vi "getShootingParameters.vi"(0 "shotTime":dbl, 1 "Turret_Angle_Deg":dbl, 2 "RobotPose":T3={"TRANSLATION"={"X"=0.0, "Y"=0.0}, "ROTATION"={"VALUE"=0.0, "COS"=1.0, "SIN"=0.0}} {"ROTATION"."SIN" format="%13.4f"; "ROTATION"."COS" format="%13.4f"; "ROTATION"."VALUE" format="%13.4f"; "TRANSLATION"."Y" format="%14.3f"; "TRANSLATION"."X" format="%14.3f"}, 3 "TurretToField":T3={"TRANSLATION"={"X"=0.0, "Y"=0.0}, "ROTATION"={"VALUE"=0.0, "COS"=1.0, "SIN"=0.0}} {"ROTATION"."SIN" format="%13.4f"; "ROTATION"."COS" format="%13.4f"; "ROTATION"."VALUE" format="%13.4f"; "TRANSLATION"."Y" format="%14.3f"; "TRANSLATION"."X" format="%14.3f"}, 5 "ShootingGoalPose":T3={"TRANSLATION"={"X"=0.0, "Y"=0.0}, "ROTATION"={"VALUE"=0.0, "COS"=1.0, "SIN"=0.0}} {"ROTATION"."SIN" format="%13.4f"; "ROTATION"."COS" format="%13.4f"; "ROTATION"."VALUE" format="%13.4f"; "TRANSLATION"."Y" format="%14.3f"; "TRANSLATION"."X" format="%14.3f"}, 6 "RobotVelocity":T1, 10 "AllowShootOnMove":bool) -> (9 "shot_speed":dbl, 11 "turret_adjustment":dbl, 13 "turret_error":T2 {"SIN" format="%13.4f"; "COS" format="%13.4f"; "VALUE" format="%13.4f"}, 14 "uncompensated_yaw_angle_deg":dbl, 15 "uncompensated_range_m":dbl, 16 "effective_yaw_angle_deg":dbl, 17 "effective_range_m":dbl, 18 "effective_yaw_feedforward_velocity_deg_s":dbl, 19 "effective_range_feedforward_m_s":dbl)   [LabVIEW 2023]
doc: "getShootingParameters is a stripped code from Team 254 - FRC_2022 repo, and re-implemented in LabVIEW.\n\nReturns the Transform2d that maps the one pose to another.\n\nParameter:\n - shotTime - Average shot time in seconds for a Game Piece traveling from robot to goal.\n - RobotPose - Current Field-To-Robot Pose.\n - Turret_Angle_Deg - Current Turret's absolute angle in degrees.\n - TurretToField - Current Turret-To-Field Pose ( from ([Robot-To-Turret] + [Field-To-Robot]).inverse )\n - ShootingGoalPose - Your Shooting Target Pose (Field-To-Goal)\n - RobotVelocity - Current ChassisSpeeds (vX, vY, vAng) but in Twist2d\n - AllowShootOnMove - Enable ShootOnMove correction\n\nReturns:\n - uncompensated_yaw_angle_deg - Yaw angle setpoint for Turret\n - uncompensated_range_m - Distance between turret and Goal\n - effective_yaw_angle_deg - (ShootOnMove) Yaw angle setpoint for Turret\n - effective_range_m - (ShootOnMove) Distance between turret and Goal\n - effective_yaw_feedforward_velocity_deg_s - FF value for velocity correction (only correction for uncompensated_yaw_angle)\n - effective_range_feedforward_m_s - FF value (TBD)"
uses:
  <vilib>/Rock Robotics/WPI/ThirdParty/JAS_Junk/TrajLib/TypeDef/POSE2D.ctl
  <vilib>/Rock Robotics/WPI/ThirdParty/JAS_Junk/TrajLib/TypeDef/TRANSLATION2D.ctl
  <vilib>/Rock Robotics/WPI/ThirdParty/JAS_Junk/TrajLib/TypeDef/ROTATION2D.ctl
  <vilib>/Rock Robotics/WPI/ThirdParty/JAS_Junk/TrajLib/TypeDef/TRANSFORM2D.ctl
  <vilib>/Rock Robotics/WPI/ThirdParty/JAS_Junk/TrajLib/TypeDef/TWIST2D.ctl
  <vilib>/Rock Robotics/WPI/ThirdParty/JAS_Junk/TrajLib/Conv_Deg_Radians.vi
  <vilib>/Rock Robotics/WPI/ThirdParty/JAS_Junk/TrajLib/Rotation2d_CreateAngle.vi
  <vilib>/Rock Robotics/WPI/ThirdParty/JAS_Junk/TrajLib/Pose2d_RelativeTo.vi
  <vilib>/Rock Robotics/WPI/ThirdParty/JAS_Junk/TrajLib/Pose2d_TransformBy.vi
  <vilib>/Rock Robotics/WPI/ThirdParty/JAS_Junk/TrajLib/Rotation2d_RotateBy.vi
  <vilib>/Rock Robotics/WPI/ThirdParty/JAS_Junk/TrajLib/Rotation2d_GetRadians.vi
  <vilib>/Rock Robotics/WPI/ThirdParty/JAS_Junk/TrajLib/Transform2d_Create_PosePose.vi
  <vilib>/Rock Robotics/WPI/ThirdParty/JAS_Junk/TrajLib/Pose2d_New_TRRO.vi
  <vilib>/Rock Robotics/WPI/ThirdParty/JAS_Junk/TrajLib/Translation2d_Plus.vi
  <vilib>/Rock Robotics/WPI/ThirdParty/JAS_Junk/TrajLib/Translation2d_Minus.vi
  <vilib>/Rock Robotics/WPI/ThirdParty/JAS_Junk/TrajLib/Rotation2d_Minus.vi
  <vilib>/Rock Robotics/WPI/ThirdParty/JAS_Junk/TrajLib/Trajectory_Library.lvlib
panel:
  out "aimingParams.robot_to_goal_rotation":T2 {"SIN" format="%13.4f"; "COS" format="%13.4f"; "VALUE" format="%13.4f"}
  out "aimingParams.range":dbl
  out "RobotToGoal_tf":T5={"TRANSLATION"={"X"=0.0, "Y"=0.0}, "ROTATION"={"VALUE"=0.0, "COS"=1.0, "SIN"=0.0}, "xF"=FALSE} {"ROTATION"."SIN" format="%13.4f"; "ROTATION"."COS" format="%13.4f"; "ROTATION"."VALUE" format="%13.4f"; "TRANSLATION"."Y" format="%14.3f"; "TRANSLATION"."X" format="%14.3f"}
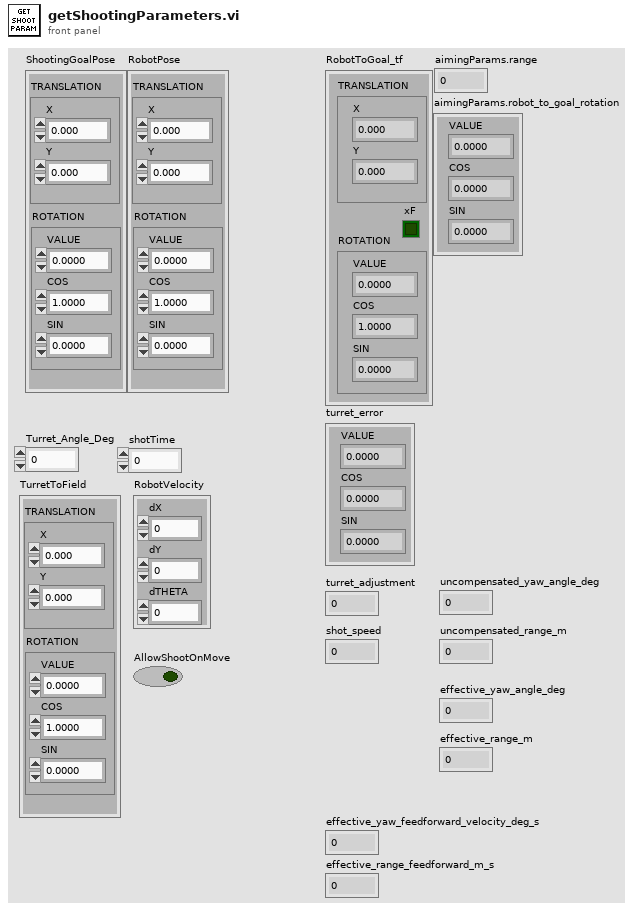
[diagram p1: front panel]
types:
  T1 = typedef "Trajectory_Library.lvlib/TWIST2D.ctl" = cluster{"dX":dbl, "dY":dbl, "dTHETA":dbl}
  T2 = typedef "Trajectory_Library.lvlib/ROTATION2D.ctl" = cluster{"VALUE":dbl, "COS":dbl, "SIN":dbl}
  T3 = typedef "Trajectory_Library.lvlib/POSE2D.ctl" = cluster{"TRANSLATION":T4, "ROTATION":T2}
  T4 = typedef "Trajectory_Library.lvlib/TRANSLATION2D.ctl" = cluster{"X":dbl, "Y":dbl}
  T5 = typedef "Trajectory_Library.lvlib/TRANSFORM2D.ctl" = cluster{"TRANSLATION":T4, "ROTATION":T2, "xF":bool}
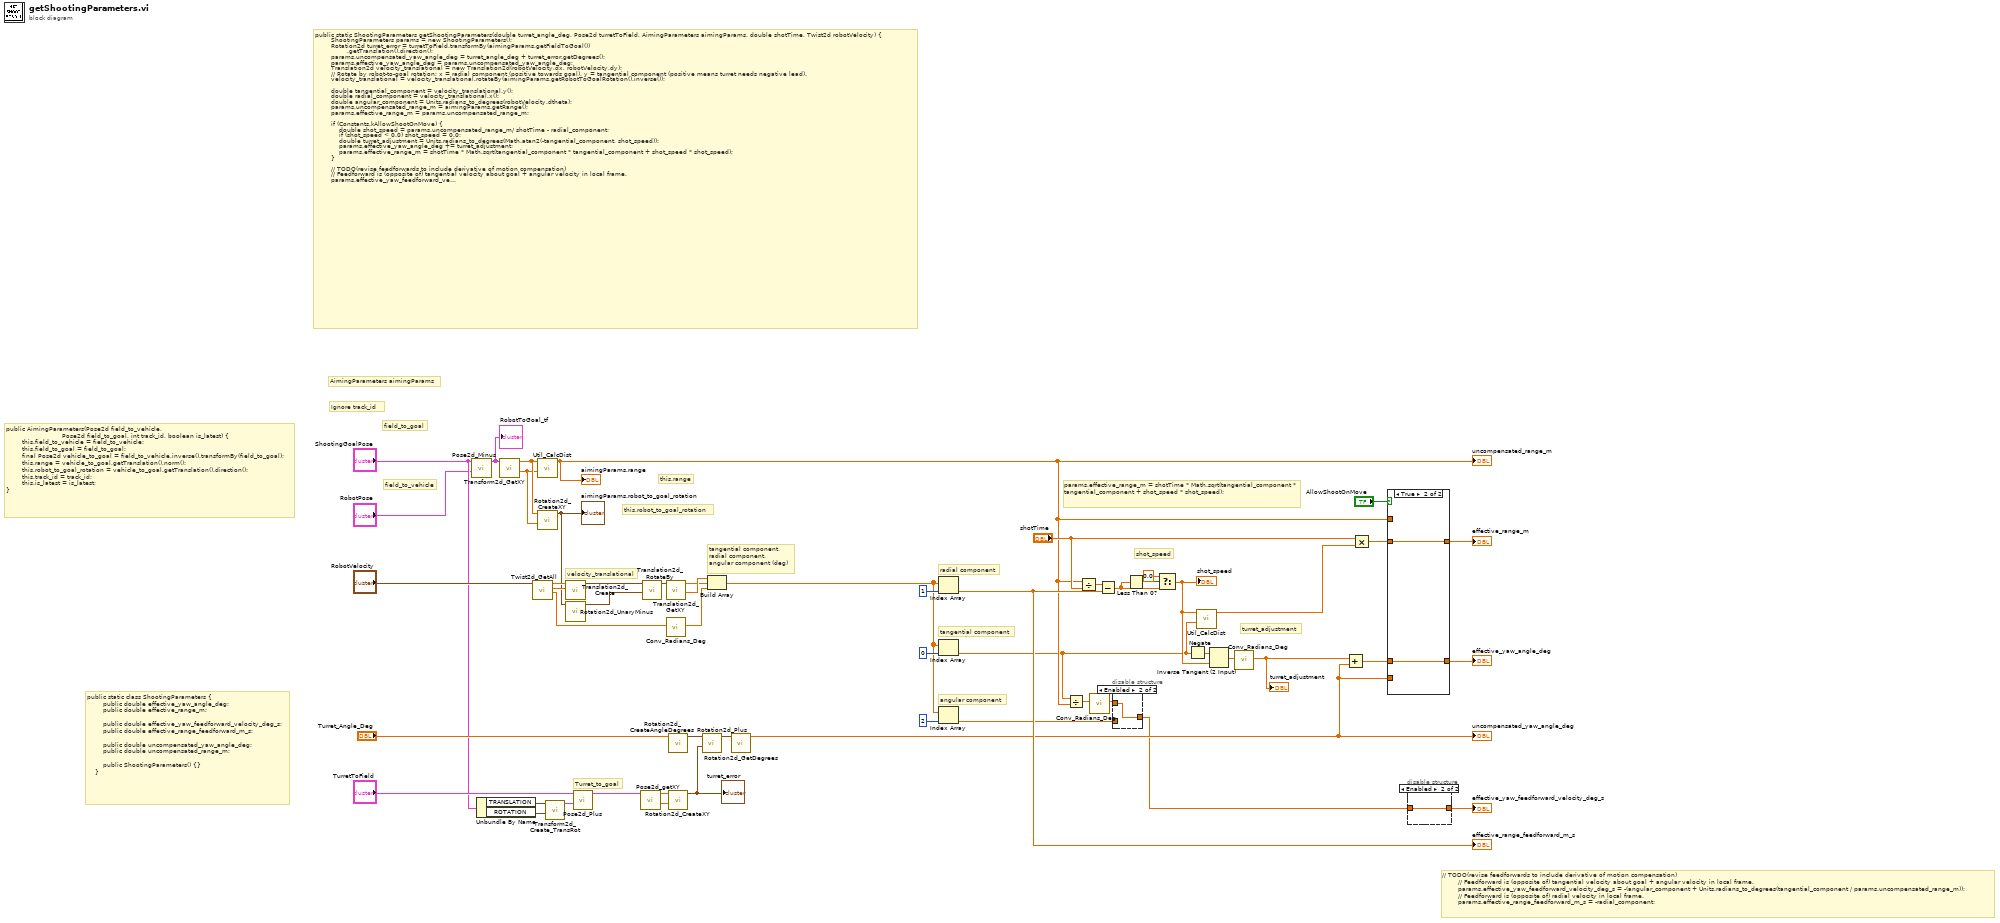
[diagram p0: block diagram]
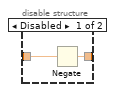
[diagram p2: hidden frame]
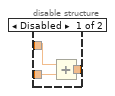
[diagram p3: hidden frame]
diagram:
  # "// TODO(revise feedforwards to include derivative of motion compensation)\n        // Feedforward is (opposite of) tangential velocity about goal + angular velocity in local frame.\n        params.effective_yaw_feedforward_velocity_deg_s = -(angular_component + Units.radians_to_degrees(tangential_component / params.uncompensated_range_m));\n        // Feedforward is (opposite of) radial velocity in local frame.\n        params.effective_range_feedforward_m_s = -radial_component;"
  # "angular component"
  # "radial component"
  # "tangential component"
  # "params.effective_range_m = shotTime * Math.sqrt(tangential_component * tangential_component + shot_speed * shot_speed);"
  # "turret_adjustment"
  # "shot_speed"
  # "tangential component,\nradial component,\nangular component (deg)"
  # "velocity_translational"
  # "Turret_to_goal"
  # "public static class ShootingParameters {\n        public double effective_yaw_angle_deg;\n        public double effective_range_m;\n\n        public double effective_yaw_feedforward_velocity_deg_s;\n        public double effective_range_feedforward_m_s;\n\n        public double uncompensated_yaw_angle_deg;\n        public double uncompensated_range_m;\n\n        public ShootingParameters() {}\n    }"
  # "public static ShootingParameters getShootingParameters(double turret_angle_deg, Pose2d turretToField, AimingParameters aimingParams, double shotTime, Twist2d robotVelocity) {\n        ShootingParameters params = new ShootingParameters();\n        Rotation2d turret_error = turretToField.transformBy(aimingParams.getFieldToGoal())\n                .getTranslation().direction();\n        params.uncompensated_yaw_angle_deg = turret_angle_deg + turret_error.getDegrees();\n        params.effective_yaw_angle_deg = params.uncompensated_yaw_angle_deg;\n        Translation2d velocity_translational = new Translation2d(robotVelocity.dx, robotVelocity.dy);\n        // Rotate by robot-to-goal rotation; x = radial component (positive towards goal), y = tangential component (positive means turret needs negative lead).\n        velocity_translational = velocity_translational.rotateBy(aimingParams.getRobotToGoalRotation().inverse());\n\n        double tangential_component = velocity_translational.y();\n        double radial_component = velocity_translational.x();\n        double angular_component = Units.radians_to_degrees(robotVelocity.dtheta);\n        params.uncompensated_range_m = aimingParams.getRange();\n        params.effective_range_m = params.uncompensated_range_m;\n\n        if (Constants.kAllowShootOnMove) {\n            double shot_speed = params.uncompensated_range_m/ shotTime - radial_component;\n            if (shot_speed < 0.0) shot_speed = 0.0;\n            double turret_adjustment = Units.radians_to_degrees(Math.atan2(-tangential_component, shot_speed));\n            params.effective_yaw_angle_deg += turret_adjustment;\n            params.effective_range_m = shotTime * Math.sqrt(tangential_component * tangential_component + shot_speed * shot_speed);\n        }\n\n        // TODO(revise feedforwards to include derivative of motion compensation)\n        // Feedforward is (opposite of) tangential velocity about goal + angular velocity in local frame.\n        params.effective_yaw_feedforward_velocity_deg_s = -(angular_component + Units.radians_to_degrees(tangential_component / params.uncompensated_range_m));\n        // Feedforward is (opposite of) radial velocity in local frame.\n        params.effective_range_feedforward_m_s = -radial_component;\n        return params;\n    }\n}"
  # "AimingParameters aimingParams"
  # "this.robot_to_goal_rotation"
  # "this.range"
  # "field_to_goal"
  # "field_to_vehicle"
  # "Ignore track_id"
  # "public AimingParameters(Pose2d field_to_vehicle,\n                            Pose2d field_to_goal, int track_id, boolean is_latest) {\n        this.field_to_vehicle = field_to_vehicle;\n        this.field_to_goal = field_to_goal;\n        final Pose2d vehicle_to_goal = field_to_vehicle.inverse().transformBy(field_to_goal);\n        this.range = vehicle_to_goal.getTranslation().norm();\n        this.robot_to_goal_rotation = vehicle_to_goal.getTranslation().direction();\n        this.track_id = track_id;\n        this.is_latest = is_latest;\n}"
  n1 = call <vilib>:"Pose2d_Minus.vi"("other POSE"="RobotPose", "in POSE"="ShootingGoalPose") -> ("outTRANSFORM"=w55:T5)  [unwired: 9 in]
  "RobotToGoal_tf" <- w55
  n2 = Unbundle By Name("ShootingGoalPose") -> ("TRANSLATION"=w51:T4, "ROTATION"=w50:T2)
  n3 = call <vilib>:"Transform2d_GetXY.vi"("inTRANSFORM"=w55) -> ("Y"=w53:dbl, "X"=w54:dbl)  [unwired: 9 in]
  n4 = call <vilib>:"Twist2d_GetAll.vi"("TWIST"="RobotVelocity") -> ("dTHETA"=w34:dbl, "dY"=w39:dbl, "dX"=w40:dbl)  [unwired: 8 in]
  n5 = call <vilib>:"Util_CalcDist.vi"("Y"=w53, "X"=w54) -> ("DIST"=w9:dbl)  [unwired: 9 in]
  "aimingParams.range" <- w9
  "uncompensated_range_m" <- w9
  n6 = call <vilib>:"Rotation2d_CreateXY.vi"("Y or sine"=w53, "X or  cosine"=w54) -> ("ROTATION"=w38:T2)  [unwired: 9 in]
  "aimingParams.robot_to_goal_rotation" <- w38
  n7 = call <vilib>:"Transform2d_Create_TransRot.vi"("ROTATION"=w50, "TRANSLATION"=w51) -> ("TRANSFORM"=w49:T5)  [unwired: 9 in]
  n8 = call <vilib>:"Translation2d_Create.vi"("Y"=w39, "X"=w40) -> ("TRANSLATION"=w37:T4)  [unwired: 9 in]
  n9 = call <vilib>:"Rotation2d_UnaryMinus.vi"("in ROTATION"=w38) -> ("out ROTATION"=w36:T2)  [unwired: 10 in]
  n10 = call <vilib>:"Pose2d_Plus.vi"("other TRANSFORM"=w49, "in POSE"="TurretToField") -> ("out POSE"=w48:T3)  [unwired: 9 in]
  n11 = call <vilib>:"Pose2d_getXY.vi"("in POSE"=w48) -> ("Y"=w46:dbl, "X"=w47:dbl)  [unwired: 9 in]
  n12 = call <vilib>:"Translation2d_RotateBy.vi"("other Rotation"=w36, "In Translation"=w37) -> ("Out Translation"=w35:T4)  [unwired: 9 in]
  n13 = call <vilib>:"Translation2d_GetXY.vi"("In Translation"=w35) -> ("Y"=w32:dbl, "X"=w31:dbl)  [unwired: 9 in]
  n14 = call <vilib>:"Conv_Radians_Deg.vi"("Radians"=w34) -> ("Degrees"=w33:dbl)  [unwired: 10 in]
  n15 = call <vilib>:"Rotation2d_CreateAngleDegrees.vi"("Angle_Degrees"="Turret_Angle_Deg") -> ("ROTATION"=w44:T2)  [unwired: 10 in]
  n16 = call <vilib>:"Rotation2d_CreateXY.vi"("Y or sine"=w46, "X or  cosine"=w47) -> ("ROTATION"=w43:T2)  [unwired: 9 in]
  "turret_error" <- w43
  n17 = call <vilib>:"Rotation2d_Plus.vi"("other ROTATION"=w43, "in ROTATION"=w44) -> ("out ROTATION"=w42:T2)  [unwired: 9 in]
  n18 = Build Array(w32, w31, w33) -> (w10:dbl[])
  n19 = call <vilib>:"Rotation2d_GetDegrees.vi"("in ROTATION"=w42) -> ("AngleDegrees"=w12:dbl)  [unwired: 10 in]
  "uncompensated_yaw_angle_deg" <- w12
  n20 = Index Array(array=w10, index=1) -> (element=w22:dbl)
  "effective_range_feedforward_m_s" <- w22
  n21 = Index Array(array=w10, index=0) -> (element=w8:dbl)
  n22 = Index Array(array=w10, index=2) -> (element=w5:dbl)
  n23 = Divide(x=w8, y=w9) -> (x/y=w7:dbl)
  n24 = Divide(x=w9, y="shotTime") -> (x/y=w30:dbl)
  n25 = call <vilib>:"Conv_Radians_Deg.vi"("Radians"=w7) -> ("Degrees"=w6:dbl)  [unwired: 10 in]
  n26 = Subtract(x=w30, y=w22) -> (x-y=w28:dbl)
  n27 = disable-structure shown="Enabled" {
    disable-tunnel: w6 -> [w58 w59]
    disable-tunnel: w5 -> [w57 _]
    disable-tunnel: [w56 w59] -> w4
    frame Disabled {
      n28 = Add(x=w58, y=w57) -> (x+y=w56:dbl)
    }
    frame Enabled {
    }
  }
  n29 = Less Than 0?(x=w28) -> (x < 0?=w29:bool)
  n30 = Select(t=0.0, s=w29, f=w28) -> (s? t:f=w19:dbl)
  "shot_speed" <- w19
  n31 = Negate(x=w8) -> (-x=w24:dbl)
  n32 = call <vilib>:"Util_CalcDist.vi"("Y"=w8, "X"=w19) -> ("DIST"=w18:dbl)  [unwired: 9 in]
  n33 = Inverse Tangent (2 Input)(1:w19, 2:w24) -> (0:w23:dbl)
  n34 = call <vilib>:"Conv_Radians_Deg.vi"("Radians"=w23) -> ("Degrees"=w21:dbl)  [unwired: 10 in]
  "turret_adjustment" <- w21
  n35 = Add(x=w21, y=w12) -> (x+y=w14:dbl)
  n36 = Multiply(x="shotTime", y=w18) -> (x*y=w16:dbl)
  n37 = case shown="True" "AllowShootOnMove" {
    tunnel: w16 -> [_ w63]
    tunnel: [w61 w63] -> w15
    tunnel: w9 -> [w61 _]
    tunnel: w14 -> [_ w62]
    tunnel: [w60 w62] -> w13
    tunnel: w12 -> [w60 _]
    frame False {
    }
    frame True {
    }
  }
  "effective_yaw_angle_deg" <- w13
  "effective_range_m" <- w15
  n38 = disable-structure shown="Enabled" {
    disable-tunnel: w4 -> [w65 w66]
    disable-tunnel: [w64 w66] -> w3
    frame Disabled {
      n39 = Negate(x=w65) -> (-x=w64:dbl)
    }
    frame Enabled {
    }
  }
  "effective_yaw_feedforward_velocity_deg_s" <- w3
